vi "EXCOM_CMD_TEST.vi"(2 "Commande #":i32=25, 7 "Args":dbl[](array[numeric]) format="%.2f", 11 "Error IN":errorcluster) -> (4 "VRN OUT":refnum<visa-resource-name>="COM4", 8 "OK Done":bool=TRUE, 15 "Error OUT":errorcluster={"status"=FALSE, "code"=1073676294, "source"="VISA Read in EXCOM_CMD_TEST.vi"})   [LabVIEW 2011]
uses:
  <vilib>/Instr/_visa.llb/VISA Configure Serial Port (Instr).vi
panel:
  in  "Close Connection ?":bool
  out "read buffer":string="   0.002869\r   9.910949\r  10.026647\r2012.500000\r   1.226672\r   9.913818\r  13.878236\r2012.748123\r 956.000000\r   0.359504\r-108.707400\r"
  in  "baud rate (9600)":u32=57600
  in  "VISA resource name":refnum<visa-resource-name>="COM4"
  out "Cmd String":string="25\r"
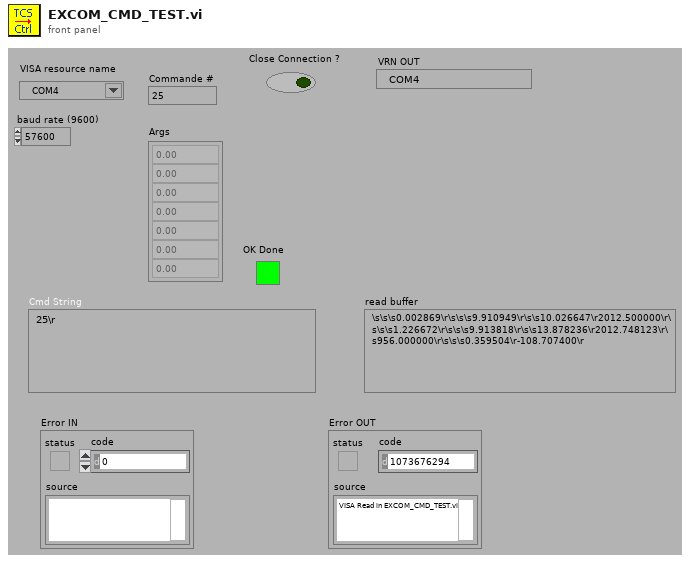
[diagram p1: front panel]
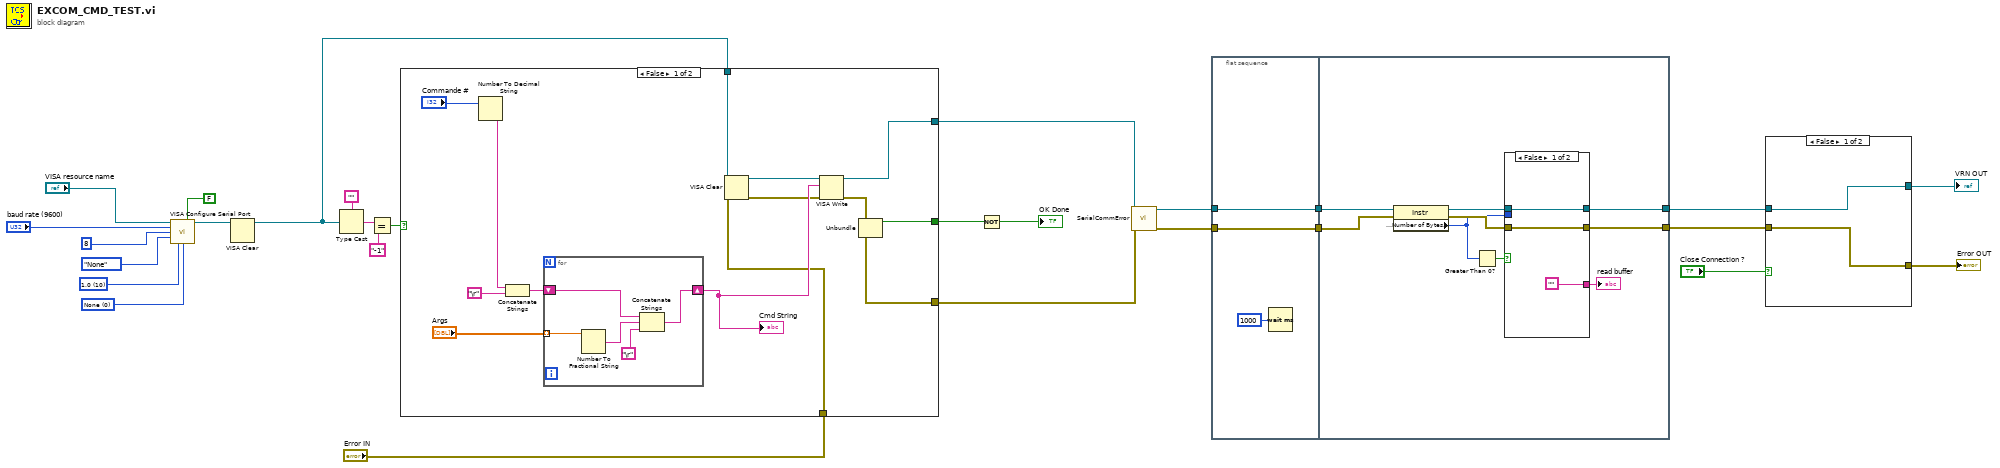
[diagram p0: block diagram]
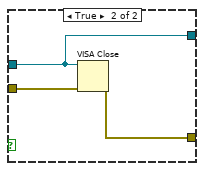
[diagram p2: hidden frame]
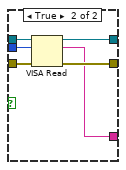
[diagram p3: hidden frame]
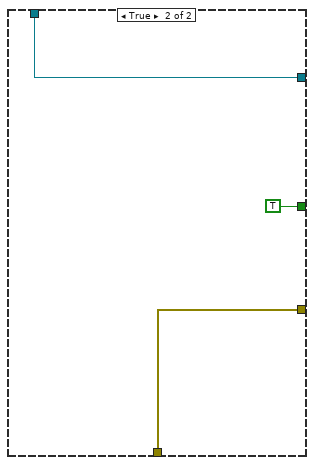
[diagram p4: hidden frame]
diagram:
  w13 = u16 0 items=["None", "XON/XOFF", "RTS/CTS", "XON/XOFF & RTS/CTS", "DTR/DSR", "XON/XOFF & DTR/DSR"] ("flow control (0:none)")
  w14 = u16 10 items=["1.0"=10, "1.5"=15, "2.0"=20] ("stop bits (10: 1 bit)")
  n1 = call-poly "VISA Configure Serial Port"("VISA resource name"="VISA resource name", "Enable Termination\nChar (T)"=FALSE ("Enable Termination\nChar (T)"), "baud rate (9600)"="baud rate (9600)", "data bits (8)"=u16 8, "parity (0:none)"=enum16{"None", "Odd", "Even", "Mark", "Space"}."None", "stop bits (10: 1 bit)"=w14, "flow control (0:none)"=w13) -> ("VISA resource name out"=w11:refnum<visa-resource-name>)  [unwired: 7 in, 1 out]
  n2 = VISA Clear(VISA resource name=w11) -> (VISA resource name out=w10:refnum<visa-resource-name>)  [unwired: 1 in, 1 out]
  n3 = Type Cast(type="", x=w10) -> (*(type *) &x=w24:string)
  n4 = Equal?(x=w24, y="-1") -> (x = y?=w22:bool)
  n5 = case shown="False" w22 {
    tunnel: [w39 TRUE ("status")] -> w26
    tunnel: w10 -> [w30 w46]
    tunnel: [w37 w47] -> w19
    tunnel: "Error IN" -> [w31 w47]
    tunnel: [w32 w46] -> w20
    frame False {
      n6 = Number To Decimal String(number="Commande #") -> (decimal integer string=w34:string)  [unwired: 1 in]
      n7 = Concatenate Strings(w34, "\r") -> (w35:string)
      n8 = for {
        shift-right: [w43] -> w38
        shift-left: w35 -> [w45]
        tunnel: "Args" -> [w42] mode=indexing
        n9 = Number To Fractional String(number=w42) -> (F-format string=w41:string)  [unwired: 3 in]
        n10 = Concatenate Strings(w45, w41, "\r") -> (w43:string)
      }
      "Cmd String" <- w38
      n11 = VISA Clear(VISA resource name=w30, error in (no error)=w31) -> (VISA resource name out=w29:refnum<visa-resource-name>, error out=w28:errorcluster)
      n12 = VISA Write(VISA resource name=w29, write buffer=w38, error in (no error)=w28) -> (VISA resource name out=w32:refnum<visa-resource-name>, error out=w37:errorcluster)  [unwired: 1 out]
      n13 = Unbundle(w37) -> ("status"=w39:bool)  [unwired: 2 out]
    }
    frame True {
    }
  }
  n14 = Not(x=w26) -> (.not. x?=→"OK Done":bool)
  n15 = call "SerialCommError.vi"("VISA IN"=w20, "error IN"=w19) -> ("VISA OUT"=w9:refnum<visa-resource-name>, "error OUT"=w8:errorcluster)  [unwired: 11 in, 1 out]
  n16 = flat-sequence {
    tunnel: w9 -> [w49]
    tunnel: w8 -> [w50]
    tunnel: [w50] -> w7
    tunnel: [w49] -> w6
    tunnel: w7 -> [w59]
    tunnel: w6 -> [w60]
    tunnel: [w56] -> w4
    tunnel: [w55] -> w5
    frame #0 {
      n17 = Wait (ms)(milliseconds to wait=u32 1000) -> ()  [unwired: 1 out]
    }
    frame #1 {
      n18 = property class="Instr"(reference=w60, error in=w59) -> (reference out=w58:refnum<visa-resource-name>, error out=w57:errorcluster, "Serial Settings:Number of Bytes at Serial Port"=w54:u32)
      n19 = Greater Than 0?(x=w54) -> (x > 0?=w53:bool)
      n20 = case shown="False" w53 {
        tunnel: w58 -> [w63 w69]
        tunnel: w57 -> [w62 w68]
        tunnel: [w63 w67] -> w56
        tunnel: [w62 w66] -> w55
        tunnel: w54 -> [_ w65]
        tunnel: ["" w64] -> w52
        frame False {
        }
        frame True {
          n21 = VISA Read(VISA resource name=w69, byte count=w65, error in (no error)=w68) -> (VISA resource name out=w67:refnum<visa-resource-name>, read buffer=w64:string, error out=w66:errorcluster)  [unwired: 1 out]
        }
      }
      "read buffer" <- w52
    }
  }
  n22 = case shown="False" "Close Connection ?" {
    tunnel: w5 -> [w70 w74]
    tunnel: w4 -> [w71 w73]
    tunnel: [w71 w73] -> w2
    tunnel: [w70 w72] -> w1
    frame False {
    }
    frame True {
      n23 = VISA Close(VISA resource name=w73, error in (no error)=w74) -> (error out=w72:errorcluster)
    }
  }
  "VRN OUT" <- w2
  "Error OUT" <- w1
